vi "subScheduler.vi"(0 "Cooling 4 Off":refnum<vi>, 1 "Cooling 3 Off":refnum<vi>, 2 "Cooling 2 Off":refnum<vi>, 3 "Cooling 1 Off":refnum<vi>, 4 "Deactivate Offset":i32=10, 5 "Activate Offset":i32=30, 6 "Cooling 4 On":refnum<vi>, 7 "Cooling 3 On":refnum<vi>, 8 "Cooling 2 On":refnum<vi>, 9 "Cooling 1 On":refnum<vi>) -> ()   [LabVIEW 2017]
panel:
  # "Upon calling, uses the offset values to create four on/off paired\nevents to use as a default cooling schedule. Uses current system\ntime. Requires timestamp references to be wired to the outputs."
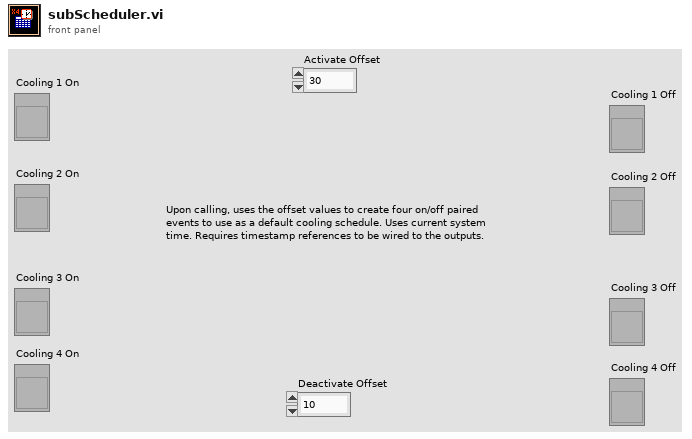
[diagram p1: front panel]
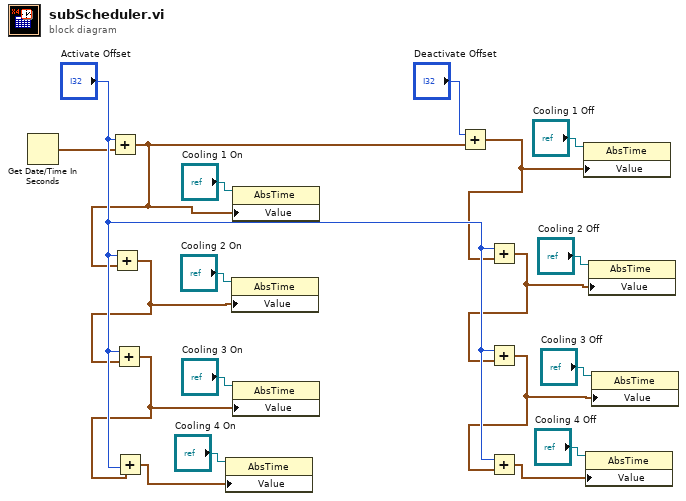
[diagram p0: block diagram]
diagram:
  n1 = Get Date/Time In Seconds() -> (seconds since 1Jan1904=w17:timestamp)
  n2 = Add(x="Activate Offset", y=w17) -> (x+y=w15:timestamp)
  n3 = Add(x="Activate Offset", y=w15) -> (x+y=w7:timestamp)
  n4 = Add(x="Activate Offset", y=w7) -> (x+y=w6:timestamp)
  n5 = Add(x="Activate Offset", y=w6) -> (x+y=w5:timestamp)
  n6 = property class="AbsTime"(reference="Cooling 4 On", "Value"=w5) -> ()  [unwired: 1 in, 2 out]
  n7 = property class="AbsTime"(reference="Cooling 2 On", "Value"=w7) -> ()  [unwired: 1 in, 2 out]
  n8 = property class="AbsTime"(reference="Cooling 1 On", "Value"=w15) -> ()  [unwired: 1 in, 2 out]
  n9 = property class="AbsTime"(reference="Cooling 3 On", "Value"=w6) -> ()  [unwired: 1 in, 2 out]
  n10 = Add(x="Deactivate Offset", y=w15) -> (x+y=w1:timestamp)
  n11 = Add(x="Activate Offset", y=w1) -> (x+y=w2:timestamp)
  n12 = Add(x="Activate Offset", y=w2) -> (x+y=w3:timestamp)
  n13 = Add(x="Activate Offset", y=w3) -> (x+y=w4:timestamp)
  n14 = property class="AbsTime"(reference="Cooling 1 Off", "Value"=w1) -> ()  [unwired: 1 in, 2 out]
  n15 = property class="AbsTime"(reference="Cooling 4 Off", "Value"=w4) -> ()  [unwired: 1 in, 2 out]
  n16 = property class="AbsTime"(reference="Cooling 2 Off", "Value"=w2) -> ()  [unwired: 1 in, 2 out]
  n17 = property class="AbsTime"(reference="Cooling 3 Off", "Value"=w3) -> ()  [unwired: 1 in, 2 out]
